vi "sub_qam_demod.vi"(8 "symbol map":cdb[](array[numeric]), 11 "symbol":cdb[](array[numeric])) -> (3 "bitstream":i16[](array[numeric]))   [LabVIEW 2014]
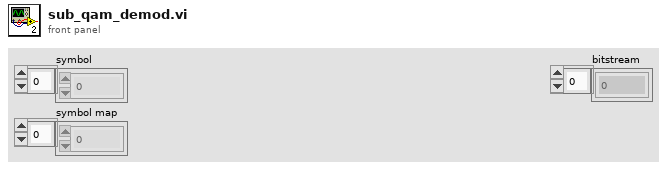
[diagram p1: front panel]
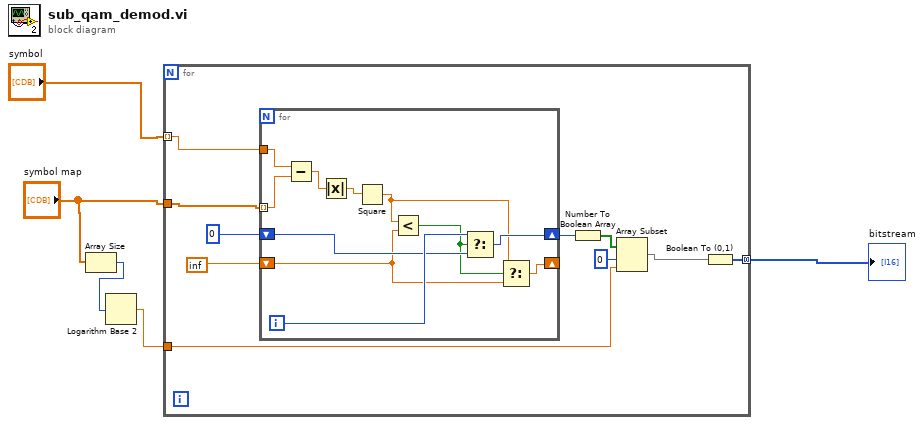
[diagram p0: block diagram]
diagram:
  n1 = Array Size(array="symbol map") -> (size(s)=w3:i32)
  n2 = Logarithm Base 2(1:w3) -> (0:w2:dbl)
  n3 = for {
    tunnel: "symbol" -> [w14] mode=indexing
    tunnel: "symbol map" -> [w15]
    tunnel: w2 -> [w8]
    tunnel: [w7] -> w1 mode=concatenating
    n4 = for {
      tunnel: w15 -> [w25] mode=indexing
      tunnel: w14 -> [w26]
      shift-right: [w20] -> w11
      shift-left: 0 -> [w21]
      shift-right: [w16] -> _
      shift-left: inf -> [w17]
      i -> [w22]
      n5 = Subtract(x=w26, y=w25) -> (x-y=w24:cdb)
      n6 = Absolute Value(x=w24) -> (abs(x)=w23:dbl)
      n7 = Square(x=w23) -> (x^2=w18:dbl)
      n8 = Less?(x=w18, y=w17) -> (x < y?=w19:bool)
      n9 = Select(t=w22, s=w19, f=w21) -> (s? t:f=w20:i32)
      n10 = Select(t=w18, s=w19, f=w17) -> (s? t:f=w16:dbl)
    }
    n11 = Number To Boolean Array(number=w11) -> (Boolean array=w10:bool[])
    n12 = Array Subset(array=w10, index=0, length=w8) -> (w6:bool[])
    n13 = Boolean To (0,1)(Boolean=w6) -> (0, 1=w7:i16[])
  }
  "bitstream" <- w1
